vi "K_S30_VISA Open Com Port.vi"(5 "RS-converter:\necho":bool=TRUE, 6 "error in (no error)":errorcluster, 7 "timeout":u32=200, 8 "Baudrate":enum16{"9600", "115200"}(ring), 9 "VISA resource name":refnum<visa-resource-name>="COM1") -> (0 "error out":errorcluster, 3 "VISA out":refnum<visa-resource-name>)   [LabVIEW 2012]
uses:
  K_S30_VISA Global.vi
panel:
  # "Configuration for the serial Port"
  # "V1.0, b.v."
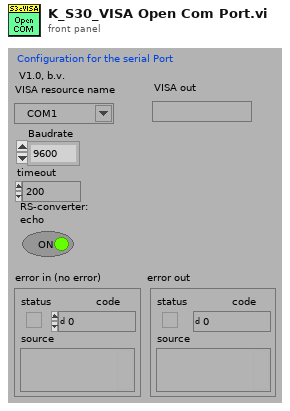
[diagram p1: front panel]
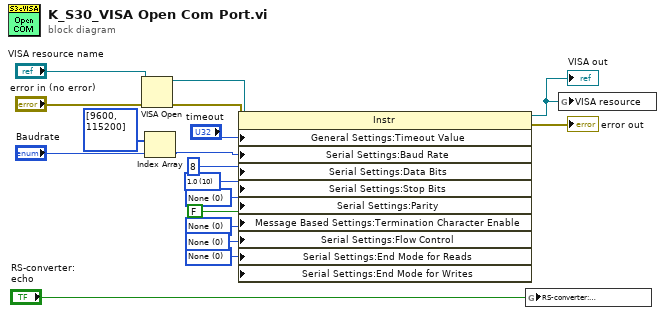
[diagram p0: block diagram]
diagram:
  w10 = u16 0 items=["None", "XON/XOFF", "RTS/CTS", "XON/XOFF & RTS/CTS", "DTR/DSR", "XON/XOFF & DTR/DSR"] ("Serial Settings:Serial Flow Control")
  w11 = u16 10 items=["1.0"=10, "1.5"=15, "2.0"=20] ("Serial Settings:Serial Stop Bits")
  w13 = u16 0 items=["None", "Odd", "Even", "Mark", "Space"] ("Serial Settings:Serial Parity")
  w15 = u16 0 items=["None", "LastBit", "TermChar"] ("Serial Settings:Serial End Mode for Reads")
  w16 = u16 0 items=["None", "LastBit", "TermChar", "Break"] ("Serial Settings:Serial End Mode for Writes")
  n1 = VISA Open(error in (no error)="error in (no error)", VISA resource name="VISA resource name") -> (VISA resource name=w7:refnum<visa-resource-name>, error out=w6:errorcluster)  [unwired: 3 in]
  n2 = Index Array(array=u32[] [9600, 115200], index="Baudrate") -> (element=w1:u32)
  n3 = property class="Instr"(reference=w7, error in=w6, "General Settings:Timeout Value"="timeout", "Serial Settings:Baud Rate"=w1, "Serial Settings:Data Bits"=u16 8 ("Serial Settings:Serial Data Bits"), "Serial Settings:Stop Bits"=w11, "Serial Settings:Parity"=w13, "Message Based Settings:Termination Character Enable"=FALSE, "Serial Settings:Flow Control"=w10, "Serial Settings:End Mode for Reads"=w15, "Serial Settings:End Mode for Writes"=w16) -> (reference out=w3:refnum<visa-resource-name>, error out=→"error out":errorcluster)
  "VISA out" <- w3
  n4 = global write "K_S30_VISA Global.vi" "RS-converter:\necho"("RS-converter:\necho") -> ()
  n5 = global write "K_S30_VISA Global.vi" "VISA resource"(w3) -> ()
